vi "AskRename.vi"(9 "Prompt":string="What is the new name?", 11 "name":string) -> (1 "OK?":bool, 3 "name 2":string caption="name")   [LabVIEW 2024]
uses:
  <vilib>/Utility/miscctls.llb/LVSelectionTypeDef.ctl
panel:
  out "error out":errorcluster
  in  "error in (no error)":errorcluster
  in  "Cancel":bool
  in  "OK":bool caption="OK2"
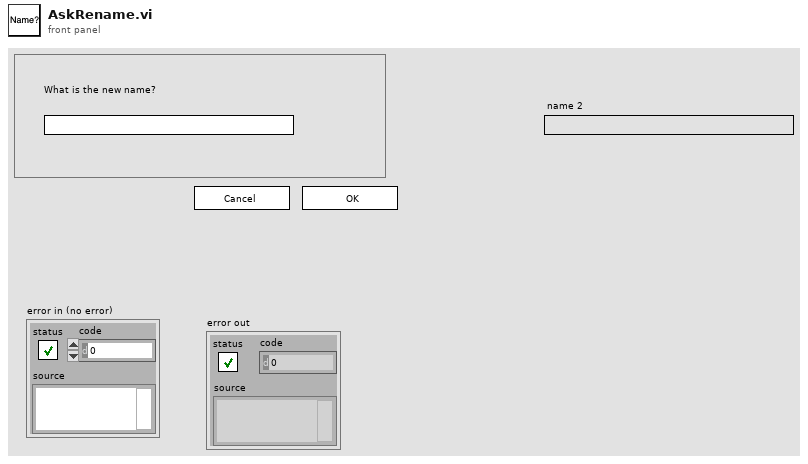
[diagram p1: front panel]
types:
  T1 = typedef "LVSelectionTypeDef.ctl" = cluster{"Selection Start":u32, "Selection End":u32}
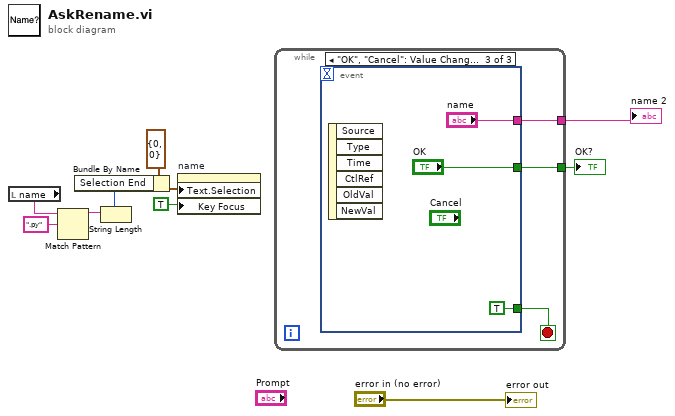
[diagram p0: block diagram]
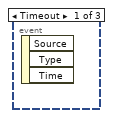
[diagram p2: hidden frame]
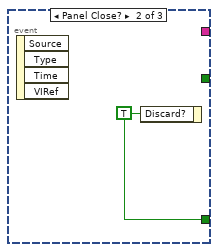
[diagram p3: hidden frame]
diagram:
  n1 = local read "name"() -> (w7:string)
  n2 = Match Pattern(string=w7, regular expression=".py") -> (before substring=w5:string)  [unwired: 1 in, 3 out]
  n3 = String Length(string=w5) -> (length=w2:i32)
  n4 = Bundle By Name(cluster=T1 {"Selection Start"=0, "Selection End"=0} ("Text.Selection"), "Selection End"=w2) -> (w3:T1)
  n5 = property on="name" class="Str"("Text.Selection"=w3, "Key Focus"=TRUE) -> ()  [unwired: 2 in, 2 out]
  n6 = while {
    tunnel: [w13] -> w8
    tunnel: [w12] -> w10
    stop <- w11 stop-if-true
    n7 = event shown="[2] \"OK\", \"Cancel\": Value Change" {
      selector: _ -> [_ _ _]
      dyn-events: _ -> [_ _ _]
      timeout: _ -> [_ _ _]
      tunnel: [_ _ "name"] -> w13
      tunnel: [_ _ "OK"] -> w12
      tunnel: [_ w14 TRUE] -> w11
      event Timeout {
        n8 = event-data() -> ()  [unwired: 1 in, 3 out]
      }
      event Panel Close? {
        w14 = TRUE ("Discard?")
        n9 = event-data() -> ()  [unwired: 1 in, 4 out]
        n10 = event-data("Discard?"=w14) -> ()  [unwired: 1 in, 1 out]
      }
      event "OK", "Cancel": Value Change {
        n11 = event-data() -> ()  [unwired: 1 in, 6 out]
      }
    }
  }
  "name 2" <- w8
  "OK?" <- w10
  "error out" <- "error in (no error)"
